vi "core_xwave2xy.vi"(7 "relative x? (F)":bool, 11 "xwave":T1={"attributes"=variant, "X"={"start"=0.0, "delta"=0.0, "units"="index", "dim"="au"}, "Y"={"data"=[], "units"="au"}}) -> (0 "x dimention":string, 1 "y units":string, 2 "x units":string, 3 "xy cluster":cluster{"X":dbl[], "Y":dbl[]})   [LabVIEW 2015]
uses:
  xwav.ctl
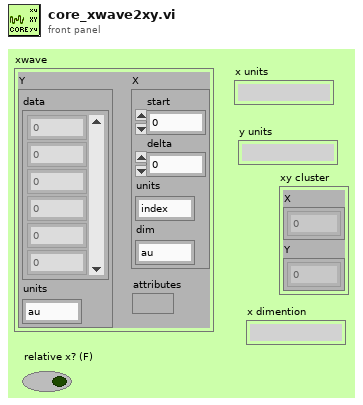
[diagram p1: front panel]
types:
  T1 = typedef "xwav.ctl" = cluster{"attributes":variant, "X":cluster{"start":dbl, "delta":dbl, "units":string, "dim":string}, "Y":cluster{"data":dbl[], "units":string}}
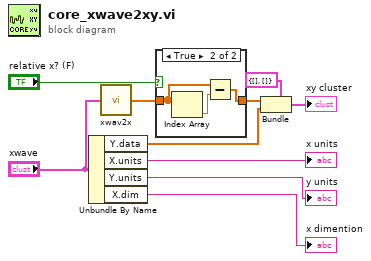
[diagram p0: block diagram]
diagram:
  n1 = Unbundle By Name("xwave") -> ("Y.data"=w10:dbl[], "X.units"=→"x units":string, "Y.units"=→"y units":string, "X.dim"=→"x dimention":string)
  n2 = call "xwav2x.vi"("xwave"="xwave") -> ("X"=w9:dbl[])  [unwired: 4 in]
  n3 = case shown="True" "relative x? (F)" {
    tunnel: w9 -> [w11 w14]
    tunnel: [w11 w12] -> w8
    frame False {
    }
    frame True {
      n4 = Index Array(array=w14) -> (element=w13:dbl)  [unwired: 1 in]
      n5 = Subtract(x=w14, y=w13) -> (x-y=w12:dbl[])
    }
  }
  n6 = Bundle(cluster=cluster{"X":dbl[], "Y":dbl[]} {"X"=[], "Y"=[]}, "X"=w8, "Y"=w10) -> (→"xy cluster":cluster{"X":dbl[], "Y":dbl[]})
